vi "Get Msg Queue.vi"(11 "Queue Msg Type Strategy in":refnum<class "Queue Msg Type Strategy.lvclass">) -> (2 "Msg Queue":refnum<queue>)   [LabVIEW 2021, in "jettl.lvlib" / "Msg Type Strategy.lvlib" / "Queue Msg Type Strategy.lvclass"]
uses:
  Queue Msg Type Strategy.lvclass
  Queue Msg Type Strategy.lvclass/Queue Msg Type Strategy.ctl
  Msg Strategy/Msg Strategy.lvclass
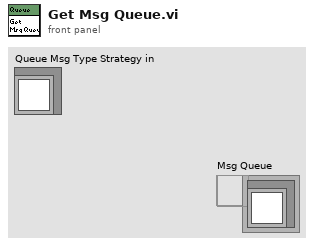
[diagram p1: front panel]
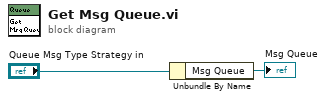
[diagram p0: block diagram]
diagram:
  n1 = Unbundle By Name("Queue Msg Type Strategy in") -> ("Msg Queue"=→"Msg Queue":refnum<queue>)
